vi "ListenPort.vi"(8 "error constant":errorcluster, 9 "StopThread":bool, 10 "IsCamera":bool, 11 "Port":u16) -> (0 "error out":errorcluster, 1 "Socket Closed":bool, 2 "OutBytes":u8[](array[numeric]), 3 "OutString":string)   [LabVIEW 2022 SP3]
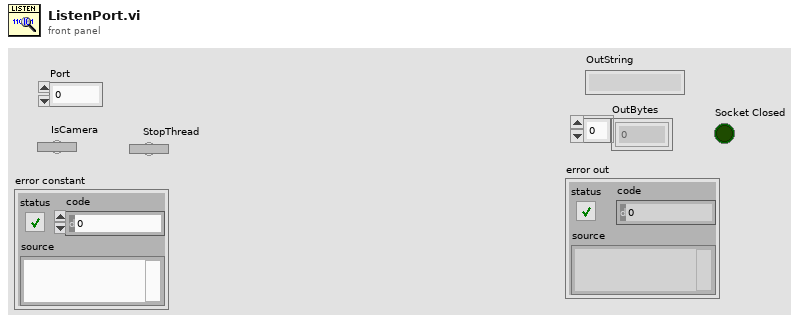
[diagram p1: front panel]
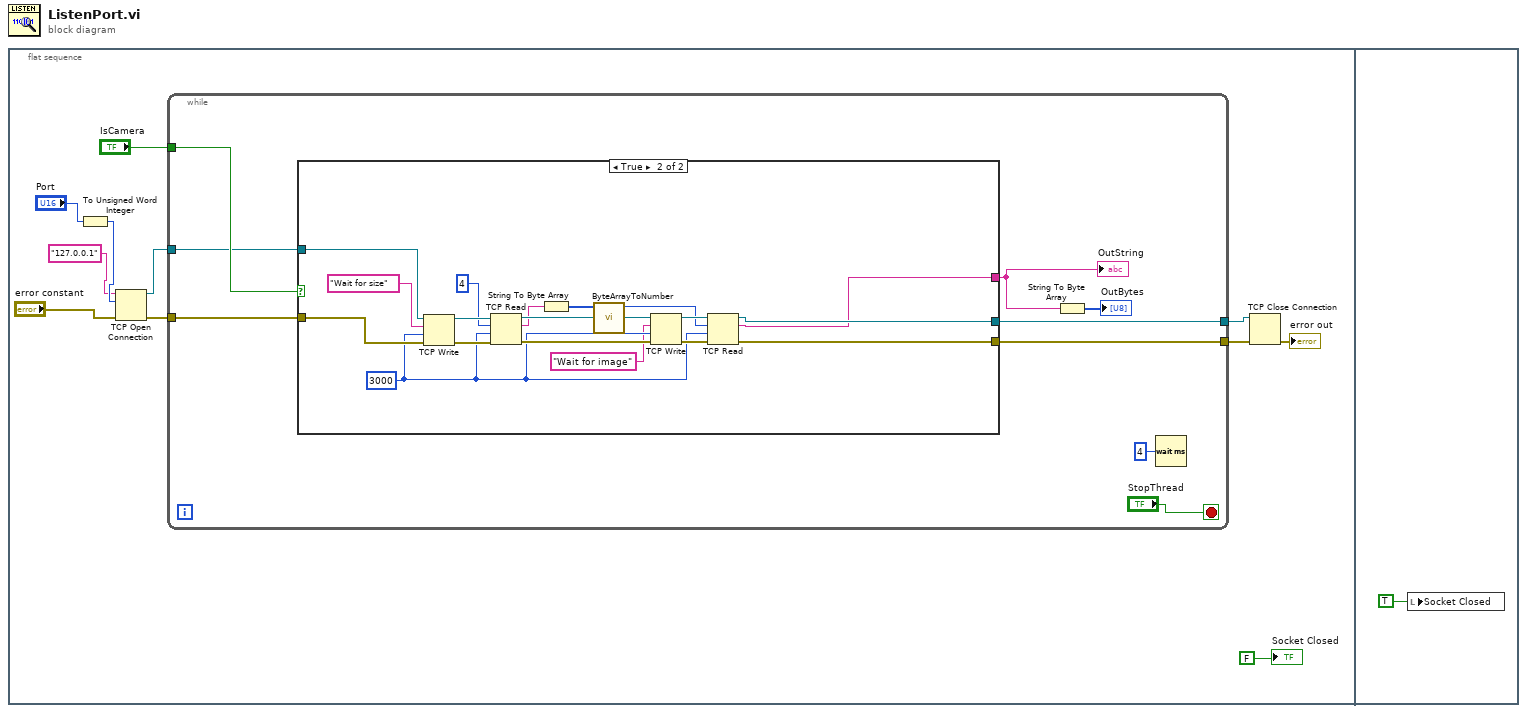
[diagram p0: block diagram]
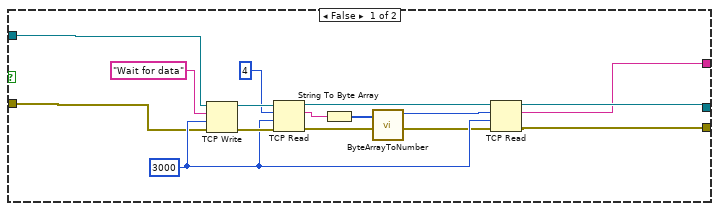
[diagram p2: hidden frame]
diagram:
  n1 = flat-sequence {
    frame #0 {
      n2 = To Unsigned Word Integer(number="Port") -> (unsigned 16bit integer=w4:u16)
      n3 = TCP Open Connection(address="127.0.0.1", remote port or service name=w4, error in (no error)="error constant") -> (connection ID=w9:refnum<k5>, error out=w7:errorcluster)  [unwired: 2 in]
      n4 = while {
        tunnel: "IsCamera" -> [w18]
        tunnel: w7 -> [w17]
        tunnel: [w16] -> w8
        tunnel: w9 -> [w14]
        tunnel: [w13] -> w10
        stop <- "StopThread" stop-if-true
        n5 = case shown="True" w18 {
          tunnel: w17 -> [w29 w52]
          tunnel: [w28 w45] -> w16
          tunnel: w14 -> [w30 w51]
          tunnel: [w24 w46] -> w13
          tunnel: [w23 w38] -> w12
          frame False {
            w32 = 3000 ("timeout ms (25000)")
            n6 = TCP Write(connection ID=w30, data in="Wait for data", error in (no error)=w29, 9:w32) -> (connection ID out=w34:refnum<k5>, error out=w35:errorcluster)  [unwired: 1 out]
            n7 = TCP Read(connection ID=w34, bytes to read=4, error in (no error)=w35, 9:w32) -> (connection ID out=w26:refnum<k5>, data out=w25:string, error out=w27:errorcluster)  [unwired: 1 in]
            n8 = String To Byte Array(string=w25) -> (unsigned byte array=w22:u8[])
            n9 = call "ByteArrayToNumber.vi"("In Array"=w22) -> ("Out Number"=w21:u32)  [unwired: 10 in]
            n10 = TCP Read(connection ID=w26, bytes to read=w21, error in (no error)=w27, 9:w32) -> (connection ID out=w24:refnum<k5>, data out=w23:string, error out=w28:errorcluster)  [unwired: 1 in]
          }
          frame True {
            w42 = 3000 ("timeout ms (25000)")
            n11 = TCP Write(connection ID=w51, data in="Wait for size", error in (no error)=w52, 9:w42) -> (connection ID out=w50:refnum<k5>, error out=w53:errorcluster)  [unwired: 1 out]
            n12 = TCP Read(connection ID=w50, bytes to read=4, error in (no error)=w53, 9:w42) -> (connection ID out=w48:refnum<k5>, data out=w40:string, error out=w43:errorcluster)  [unwired: 1 in]
            n13 = String To Byte Array(string=w40) -> (unsigned byte array=w37:u8[])
            n14 = call "ByteArrayToNumber.vi"("In Array"=w37) -> ("Out Number"=w36:u32)  [unwired: 10 in]
            n15 = TCP Write(connection ID=w48, data in="Wait for image", error in (no error)=w43, 9:w42) -> (connection ID out=w47:refnum<k5>, error out=w44:errorcluster)  [unwired: 1 out]
            n16 = TCP Read(connection ID=w47, bytes to read=w36, error in (no error)=w44, 9:w42) -> (connection ID out=w46:refnum<k5>, data out=w38:string, error out=w45:errorcluster)  [unwired: 1 in]
          }
        }
        "OutString" <- w12
        n17 = String To Byte Array(string=w12) -> (unsigned byte array=→"OutBytes":u8[])
        n18 = Wait (ms)(milliseconds to wait=u32 4) -> ()  [unwired: 1 out]
      }
      n19 = TCP Close Connection(connection ID=w10, error in (no error)=w8) -> (error out=→"error out":errorcluster)  [unwired: 1 in, 1 out]
      "Socket Closed" <- FALSE
    }
    frame #1 {
      n20 = local write "Socket Closed"(TRUE) -> ()
    }
  }
